vi "toGPS-Epoch.vi"(11 "Epoch in":refnum<class "Epoch.UTC.lvclass">) -> (2 "GPS Epoch Time":i64)   [LabVIEW 2013]
uses:
  Epoch.UTC.lvclass
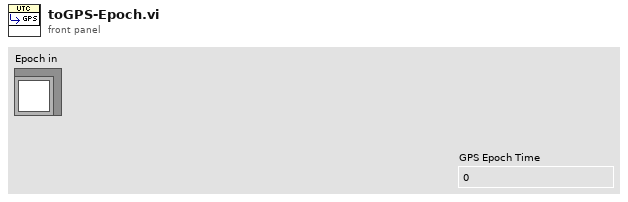
[diagram p1: front panel]
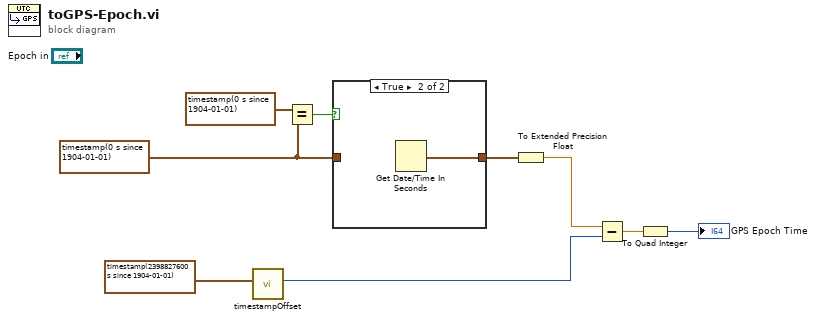
[diagram p0: block diagram]
diagram:
  w1 = timestamp(0 s since 1904-01-01) ("x")
  n1 = call "timestampOffset.vi"("Reference Time"=timestamp(2398827600 s since 1904-01-01) ("Timestamp")) -> ("Timestamp Offset"=w5:i64)  [unwired: 10 in]
  n2 = Equal?(x=timestamp(0 s since 1904-01-01), y=w1) -> (x = y?=w3:bool)
  n3 = case shown="True" w3 {
    tunnel: [w10 w11] -> w2
    tunnel: w1 -> [w10 _]
    frame False {
    }
    frame True {
      n4 = Get Date/Time In Seconds() -> (seconds since 1Jan1904=w11:timestamp)
    }
  }
  n5 = To Extended Precision Float(1:w2) -> (0:w7:ext)
  n6 = Subtract(x=w7, y=w5) -> (x-y=w9:ext)
  n7 = To Quad Integer(1:w9) -> (0:→"GPS Epoch Time":i64)
